vi "Simple Types.vi"() -> ()   [LabVIEW 2011]
uses:
  LV JSON.lvlib
panel:
  out "Cluster 2 OK?":bool
  out "Cluster 2":cluster{"abc":cluster{"def":dbl}, "jkl":dbl}
  in  "Cluster 2":cluster{"abc":cluster{"def":dbl}, "jkl":dbl}={"abc"={"def"=1.0}, "jkl"=3.0}
  out "Cluster 2 JSON":string
  out "Mismatch":bool
  out "Variant Data String":string
  out "Double out":dbl
  out "Double JSON":string
  out "Double Valid?":bool
  out "Valid?":bool
  out "String JSON":string
  out "String out":string
  in  "U32":u32
  in  "I32":i32
  in  "Single":sgl
  in  "Double":dbl=9.0
  in  "String":string="9"
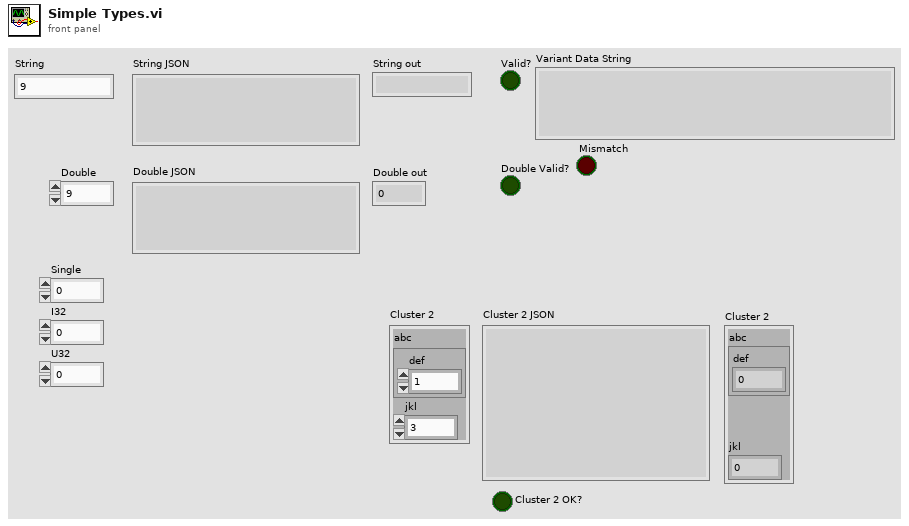
[diagram p1: front panel]
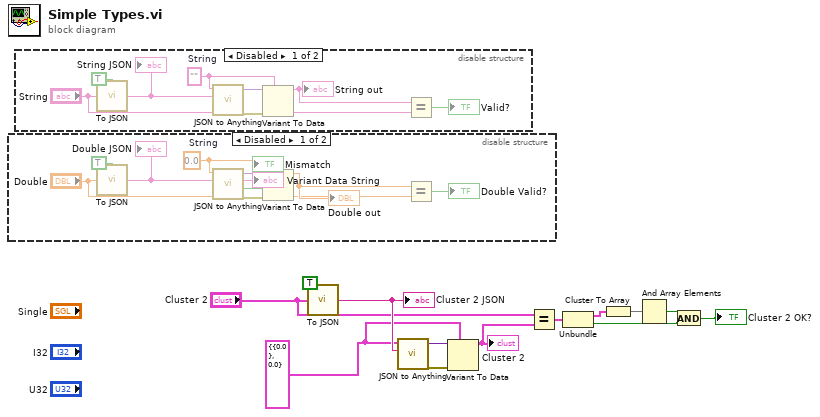
[diagram p0: block diagram]
diagram:
  w1 = cluster{"abc":cluster{"def":dbl}, "jkl":dbl} {"abc"={"def"=0.0}, "jkl"=0.0} ("Cluster 2")
  (unwired) TRUE ("Pretty Print (F)")
  n1 = disable-structure shown="Disabled" {
    frame Disabled {
      w20 = 0.0  # String
      n2 = call "To JSON.vi"("Anything"="Double", "Pretty Print (F)"=TRUE) -> ("JSON"=w19:string)
      "Double JSON" <- w19
      n3 = call "JSON to Anything.vi"("JSON Object"=w19, "Type"=w20) -> ("error out"=w17:errorcluster, "Mismatch"=→"Mismatch":bool, "Variant Data String"=→"Variant Data String":string, "Variant"=w18:variant)  [unwired: 6 in]
      n4 = Variant To Data(error in=w17, type=w20, Variant=w18) -> (data=w21:dbl)  [unwired: 1 out]
      "Double out" <- w21
      n5 = Equal?(x=w21, y="Double") -> (x = y?=→"Double Valid?":bool)
    }
    frame Enabled {
    }
  }
  n6 = disable-structure shown="Disabled" {
    frame Disabled {
      w26 = ""  # String
      n7 = call "To JSON.vi"("Anything"="String", "Pretty Print (F)"=TRUE) -> ("JSON"=w27:string)
      "String JSON" <- w27
      n8 = call "JSON to Anything.vi"("JSON Object"=w27, "Type"=w26) -> ("error out"=w29:errorcluster, "Variant"=w28:variant)  [unwired: 6 in, 2 out]
      n9 = Variant To Data(error in=w29, type=w26, Variant=w28) -> (data=w25:string)  [unwired: 1 out]
      "String out" <- w25
      n10 = Equal?(x=w25, y="String") -> (x = y?=→"Valid?":bool)
    }
    frame Enabled {
    }
  }
  n11 = call "To JSON.vi"("Anything"="Cluster 2") -> ("JSON"=w7:string)  [unwired: 1 in]
  "Cluster 2 JSON" <- w7
  n12 = call "JSON to Anything.vi"("JSON Object"=w7, "Type"=w1) -> ("error out"=w12:errorcluster, "Variant"=w11:variant)  [unwired: 6 in, 2 out]
  n13 = Variant To Data(error in=w12, type=w1, Variant=w11) -> (data=w8:cluster{"abc":cluster{"def":dbl}, "jkl":dbl})  [unwired: 1 out]
  "Cluster 2" <- w8
  n14 = Equal?(x="Cluster 2", y=w8) -> (x = y?=w9:cluster{"abc":cluster{"def":bool}, "jkl":bool})
  n15 = Unbundle(w9) -> ("abc"=w4:cluster{"def":bool}, "jkl"=w5:bool)
  n16 = Cluster To Array(cluster=w4) -> (array=w3:bool[])
  n17 = And Array Elements(Boolean array=w3) -> (logical AND=w10:bool)
  n18 = And(x=w10, y=w5) -> (x .and. y?=→"Cluster 2 OK?":bool)
